vi "Moyenne.vi"(1 "DBL-Array":sgl[](array[numeric])) -> (0 "Moyenne":sgl)   [LabVIEW 2011]
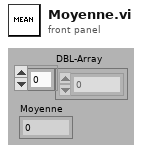
[diagram p1: front panel]
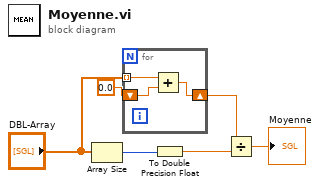
[diagram p0: block diagram]
diagram:
  n1 = Array Size(array="DBL-Array") -> (size(s)=w4:i32)
  n2 = for {
    tunnel: "DBL-Array" -> [w8] mode=indexing
    shift-right: [w9] -> w2
    shift-left: 0.0 -> [w7]
    n3 = Add(x=w8, y=w7) -> (x+y=w9:dbl)
  }
  n4 = To Double Precision Float(number=w4) -> (double precision float=w3:dbl)
  n5 = Divide(x=w2, y=w3) -> (x/y=→"Moyenne":dbl)
